vi "RSZVB Set Virtual Transform Port Pair State.vi"(6 "State (Off)":bool, 7 "Port Pair (1)":i32=1, 8 "error in (no error)":errorcluster {"code" format="%.0x"}, 9 "Function Type (Deembedding)":i32(ring) items=["Deembedding", "Embedding"], 10 "Channel (1)":i32=1, 11 "VISA session":refnum<visa-resource-name>) -> (0 "error out":errorcluster {"code" format="%.0x"}, 3 "dup VISA session":refnum<visa-resource-name>)   [LabVIEW 2011]
doc: "This VI enables or disables the deembedding/embedding VI for for port pairs.\n\nRemote-control command(s):\nCALCulate<Ch>:TRANsform:VNETworks:PPAir:DEEMbedding<List_idx>[:STATe] <Boolean> \nCALCulate<Ch>:TRANsform:VNETworks:PPAir:EMBedding<List_idx>[:STATe] <Boolean>"
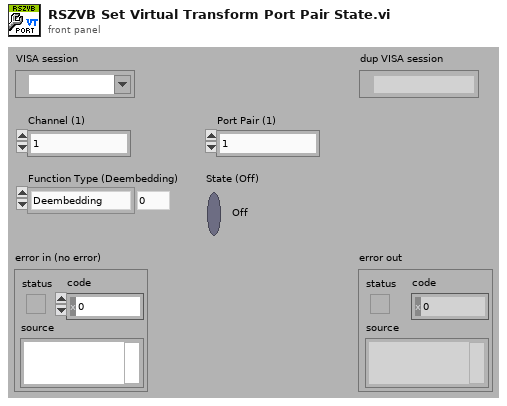
[diagram p1: front panel]
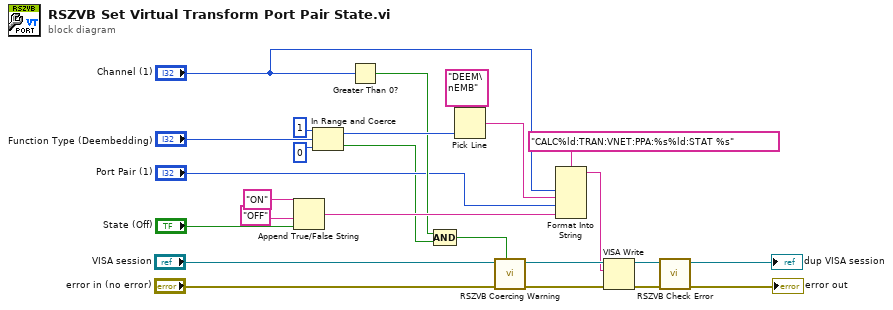
[diagram p0: block diagram]
diagram:
  n1 = Append True/False String(1:"State (Off)", 2:"OFF", 3:"ON") -> (0:w18:string)  [unwired: 1 in]
  n2 = In Range and Coerce(upper limit=1 ("lower limit"), x="Function Type (Deembedding)", lower limit=0) -> (coerced(x)=w16:i32, In Range?=w7:bool)
  n3 = Greater Than 0?(x="Channel (1)") -> (x > 0?=w14:bool)
  n4 = Compound Arithmetic op=AND(w14, w7) -> (w8:bool)
  n5 = Pick Line(multi-line string="DEEM\nEMB", line index=w16) -> (output string=w15:string)  [unwired: 1 in]
  n6 = call "RSZVB Coercing Warning.vi"("In Range?"=w8, "error in (no error)"="error in (no error)", "VISA session"="VISA session") -> ("error out"=w4:errorcluster, "dup VISA session"=w25:refnum<visa-resource-name>)  [unwired: 7 in]
  n7 = Format Into String(format string="CALC%ld:TRAN:VNET:PPA:%s%ld:STAT %s", "Channel (1)", w15, "Port Pair (1)", w18) -> (resulting string=w1:string)  [unwired: 2 in, 1 out]
  n8 = VISA Write(VISA resource name=w25, write buffer=w1, error in (no error)=w4) -> (VISA resource name out=w24:refnum<visa-resource-name>, error out=w3:errorcluster)  [unwired: 1 out]
  n9 = call "RSZVB Check Error.vi"("error in (no error)"=w3, "VISA session"=w24) -> ("error out"=→"error out":errorcluster, "dup VISA session"=→"dup VISA session":refnum<visa-resource-name>)  [unwired: 8 in]
